vi "Launcher Views.vi"(8 "error in (no error)":errorcluster, 11 "Controller in":refnum<class "Controller.lvclass">) -> (0 "error out":errorcluster, 3 "Controller out":refnum<class "Controller.lvclass">)   [LabVIEW 2020, in "Controller.lvlib" / "Controller.lvclass"]
uses:
  Controller.lvclass
  Views/[V] Main UI/[V] Main UI/[V] Main UI.lvclass
  C:/Program Files (x86)/National Instruments/LabVIEW 2020/vi.lib/ActorFramework/Actor/Actor.lvclass
  Depden On/Abstruct View/Abstruct View/Abstruct View.lvclass/Abstruct View.ctl
  Depden On/MVVM Framework/MVVM Abstruct Controller/MVVM Abstruct Controller/MVVM Abstruct Controller.lvclass/MVVM Abstruct Controller.ctl
  <vilib>/ActorFramework/Message Enqueuer/Message Enqueuer.lvclass/Message Enqueuer.ctl
  Depden On/Abstruct View/Abstruct View/Data Accessors/Write FP.Title.vi
  Depden On/MVVM Framework/MVVM Abstruct Controller/MVVM Abstruct Controller/Accessor/Read ActorMap-Views.vi
  <vilib>/ActorFramework/Message Enqueuer/Enqueue.vi
  Depden On/Abstruct View/Abstruct View Messages/Show Front Msg/Show Front Msg.lvclass
  C:/Program Files (x86)/National Instruments/LabVIEW 2020/vi.lib/ActorFramework/Message/Message.lvclass
  <vilib>/ActorFramework/Message Priority Queue/Priority Enqueue.vi
  Depden On/ActorMap/ActorMap.lvclass
  Depden On/MVVM Framework/MVVM Abstruct Controller/MVVM Abstruct Controller/MVVM Abstruct Controller.lvclass
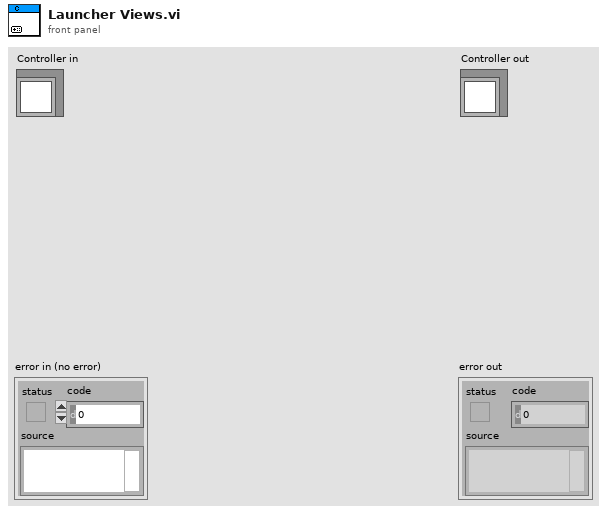
[diagram p1: front panel]
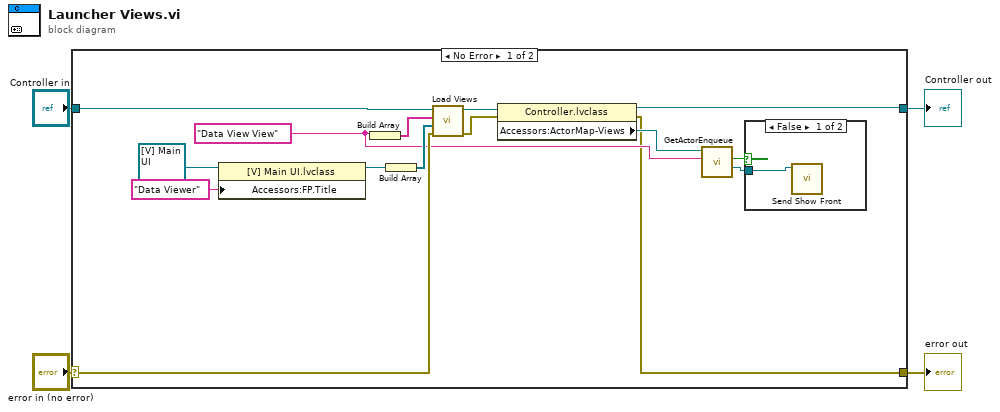
[diagram p0: block diagram]
diagram:
  n1 = case shown="No Error" "error in (no error)" {
    selector: "error in (no error)" -> [w13 w22]
    tunnel: [w5 w22] -> w3
    tunnel: [w11 w21] -> w1
    tunnel: "Controller in" -> [w19 w21]
    frame No Error {
      w9 = "Data View View" ("FP.Title")
      n2 = property class="[V] Main UI.lvclass"(reference=refnum<class "[V] Main UI.lvclass"> refnum ("[V] Main UI.lvlib:[V] Main UI.lvclass"), "Accessors:FP.Title"="Data Viewer" ("FP.Title")) -> (reference out=w16:refnum<class "[V] Main UI.lvclass">)  [unwired: 1 in, 1 out]
      n3 = Build Array(w9) -> (w14:string[])
      n4 = Build Array(w16) -> (w15:refnum<class "[V] Main UI.lvclass">[])
      n5 = call "Load Views.vi"("error in (no error)"=w13, "Views"=w15, "Names"=w14, "MVVM Abstruct Controller in"=w19) -> ("error out"=w6:errorcluster, "MVVM Abstruct Controller out"=w12:refnum<class "Controller.lvclass">)  [unwired: 6 in]
      n6 = property class="Controller.lvclass"(reference=w12, error in=w6) -> (reference out=w11:refnum<class "Controller.lvclass">, error out=w5:errorcluster, "Accessors:ActorMap-Views"=w10:refnum<class "ActorMap.lvclass">)
      n7 = call "GetActorEnqueue.vi"("name"=w9, "ActorMap in"=w10) -> ("Enqueue"=w7:refnum<class "Message Enqueuer.lvclass">, "key not found?"=w8:bool)  [unwired: 6 in, 2 out]
      n8 = case shown="False" w8 {
        tunnel: w7 -> [w20 _]
        frame False {
          n9 = call "Send Show Front.vi"("Message Enqueuer"=w20) -> ()  [unwired: 9 in, 2 out]
        }
        frame True {
        }
      }
    }
    frame Error {
    }
  }
  "error out" <- w3
  "Controller out" <- w1
